vi "num_str_remove_zero.vi"(11 "in":string="10.005000") -> (3 "out":string)   [LabVIEW 2019, in "User lib.lvlib"]
uses:
  User lib.lvlib
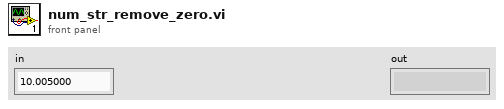
[diagram p1: front panel]
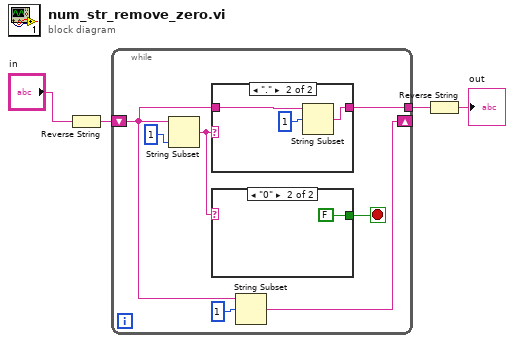
[diagram p0: block diagram]
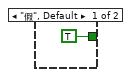
[diagram p3: hidden frame]
diagram:
  n1 = Reverse String(1:"in") -> (0:w1:string)
  n2 = while {
    shift-right: [w7] -> _
    shift-left: w1 -> [w5]
    tunnel: [w8] -> w4
    stop <- w10 stop-if-true
    n3 = String Subset(string=w5, length (rest)=1 ("长度（剩余）")) -> (substring=w9:string)  [unwired: 1 in]
    n4 = case shown="\".\"" w9 {
      tunnel: w5 -> [w12 w15]
      tunnel: [w12 w13] -> w8
      frame "假", Default {
      }
      frame "." {
        n5 = String Subset(string=w15, offset (0)=1 ("偏移量(0)")) -> (substring=w13:string)  [unwired: 1 in]
      }
    }
    n6 = case shown="\"0\"" w9 {
      tunnel: [TRUE FALSE] -> w10
      frame "假", Default {
      }
      frame "0" {
      }
    }
    n7 = String Subset(string=w5, offset (0)=1 ("偏移量(0)")) -> (substring=w7:string)  [unwired: 1 in]
  }
  n8 = Reverse String(1:w4) -> (0:→"out":string)
